vi "fgt get sensor Unit.vi"(8 "error in (no error)":errorcluster, 11 "sensorIndex":u32) -> (0 "error out":errorcluster, 3 "unit out":T1)   [LabVIEW 2020, in "fgt_SDK.lvlib"]
doc: "Get current unit on selected sensor device, default value is \"µl/min\" for flowunits and 'mbar' for pressure sensors.\nEvery sensor read value and regulation command use this unit."
uses:
  fgt_SDK.lvlib
  TypeDefs/fgt_SENSOR_UNIT.ctl
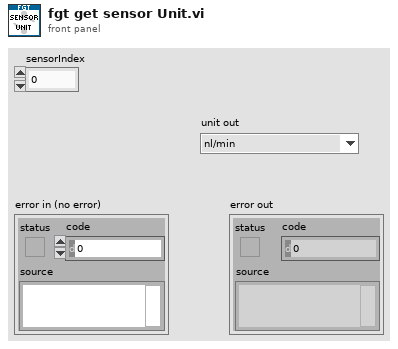
[diagram p1: front panel]
types:
  T1 = typedef "fgt_SDK.lvlib/fgt_SENSOR_UNIT.ctl" = enum16{"nl/min", "µl/s", "µl/min", "ul/h", "ml/min", "ml/h", "mbar", "kPa", "bar"}
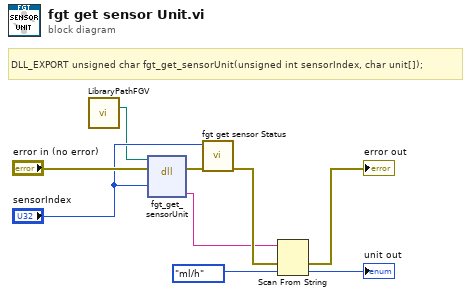
[diagram p0: block diagram]
diagram:
  # "DLL_EXPORT unsigned char fgt_get_sensorUnit(unsigned int sensorIndex, char unit[]);"
  n1 = call "LibraryPathFGV.vi"() -> ("Path Out"=w1:path)  [unwired: 14 in, 1 out]
  n2 = dll-call lib="C:/Workspace/fgt-SDK/LabVIEW/dlls/fgt_SDK_*.*" fn="fgt_get_sensorUnit"(path in=w1, error in="error in (no error)", "sensorIndex"="sensorIndex") -> (error out=w8:errorcluster, "unit"=w2:string)  [unwired: 4 in, 1 out]
  n3 = call "fgt get sensor Status.vi"("error in (no error)"=w8, "pressureIndex"="sensorIndex") -> ("error out"=w4:errorcluster)  [unwired: 9 in]
  n4 = Scan From String(input string=w2, error in=w4, default 1=fgt_SENSOR_UNIT."ml/h" ("unit out")) -> (error out=→"error out":errorcluster, output 1=→"unit out":T1)  [unwired: 2 in, 2 out]
